vi "Read Ctl Refnum.vi"(8 "error in (no error)":errorcluster, 11 "Refnum Value Source in":refnum<class "Ctrl Refnum Value Source.lvclass">) -> (0 "error out":errorcluster, 2 "Ctl Refnum":refnum<vi>, 3 "Refnum Value Source out":refnum<class "Ctrl Refnum Value Source.lvclass">)   [LabVIEW 2020, in "Composed Columns.lvlib" / "Ctrl Refnum Value Source.lvclass"]
uses:
  Ctrl Refnum Value Source.lvclass
  Ctrl Refnum Value Source.lvclass/Ctrl Refnum Value Source.ctl
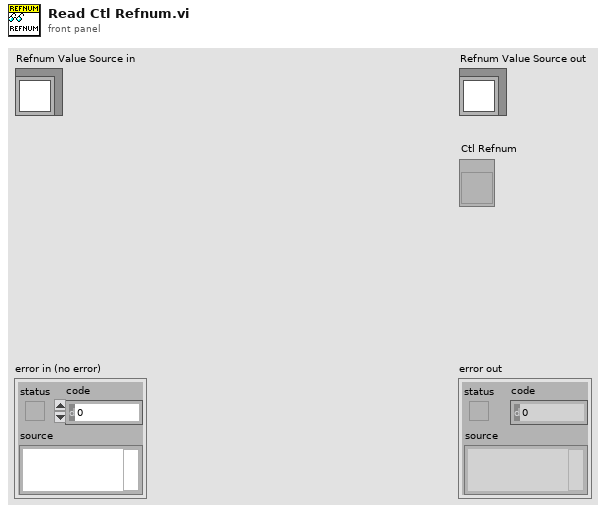
[diagram p1: front panel]
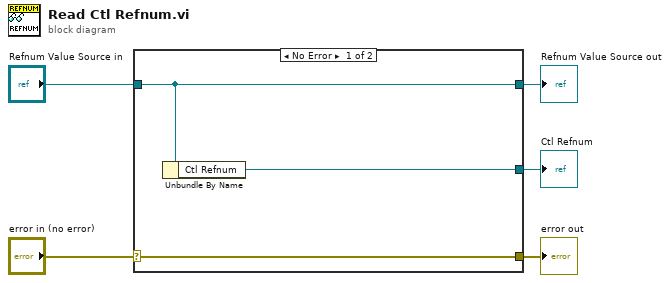
[diagram p0: block diagram]
diagram:
  n1 = case shown="No Error" "error in (no error)" {
    selector: "error in (no error)" -> [w8 w9]
    tunnel: [w8 w9] -> w4
    tunnel: [w7 w10] -> w2
    tunnel: "Refnum Value Source in" -> [w7 w10]
    tunnel: [w6 _] -> w1
    frame No Error {
      n2 = Unbundle By Name(w7) -> ("Ctl Refnum"=w6:refnum<vi>)
    }
    frame Error {
    }
  }
  "error out" <- w4
  "Refnum Value Source out" <- w2
  "Ctl Refnum" <- w1
